vi "Convert Joystick Axis to Square.vi"(11 "Joystick Axis":dbl) -> (3 "Squared":dbl)   [LabVIEW 2014]
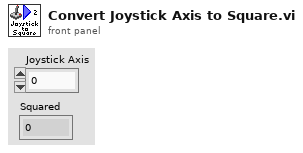
[diagram p1: front panel]
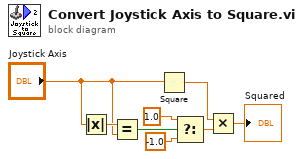
[diagram p0: block diagram]
diagram:
  n1 = Absolute Value(x="Joystick Axis") -> (abs(x)=w7:dbl)
  n2 = Equal?(x=w7, y="Joystick Axis") -> (x = y?=w8:bool)
  n3 = Square(x="Joystick Axis") -> (x^2=w5:dbl)
  n4 = Select(t=1.0, s=w8, f=-1.0) -> (s? t:f=w4:dbl)
  n5 = Multiply(x=w5, y=w4) -> (x*y=→"Squared":dbl)
